vi "Destroy.vi"(0 "reference in":refnum<class "RedisConnection.lvclass">, 11 "Error In":errorcluster) -> (4 "reference out":refnum<class "RedisConnection.lvclass">, 15 "Error Out":errorcluster)   [LabVIEW 2020, in "RedisConnection.lvclass"]
uses:
  RedisConnection.lvclass
  RedisConnection.lvclass/RedisConnection.ctl
  Ping.vi
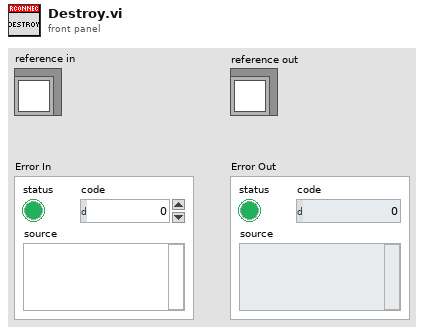
[diagram p1: front panel]
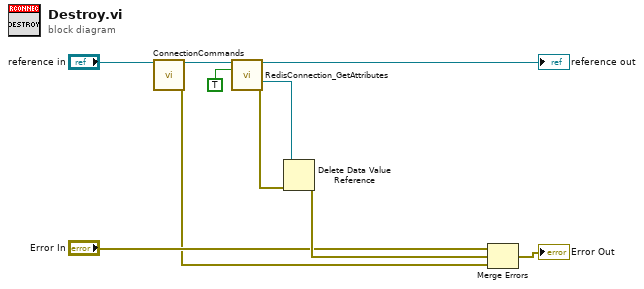
[diagram p0: block diagram]
diagram:
  n1 = call-poly "ConnectionCommands.vi"("reference in"="reference in") -> ("reference out"=w2:refnum<class "RedisConnection.lvclass">, "Error Out"=w1:errorcluster)  [unwired: 12 in, 1 out]
  n2 = call "RedisConnection_GetAttributes.vi"("reference in"=w2, "OnlyGetDvrReference(False)"=TRUE) -> ("reference out"=→"reference out":refnum<class "RedisConnection.lvclass">, "DataRef"=w7:refnum<data-value>, "Error Out"=w8:errorcluster)  [unwired: 10 in, 1 out]
  n3 = Delete Data Value Reference(data value reference=w7, error in=w8) -> (error out=w6:errorcluster)  [unwired: 1 out]
  n4 = Merge Errors("Error In", w6, w1) -> (→"Error Out":errorcluster)
